vi "Check validate frequencies.vi"(8 "Check Delta Amplitude":bool[](array[boolean]), 9 "Check Amplitude":bool[](array[boolean]), 11 "Frequencies Array":dbl[](array[numeric])) -> (0 "variance":dbl format="%0.2f", 1 "Standard deviation %":dbl, 2 "standard deviation":dbl format="%0.2f", 3 "Mean frequency":dbl format="%0.2f")   [LabVIEW 2014]
uses:
  <vilib>/Analysis/NI_AALBase.lvlib
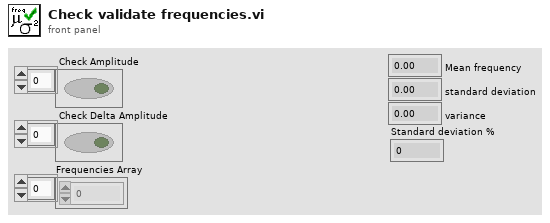
[diagram p1: front panel]
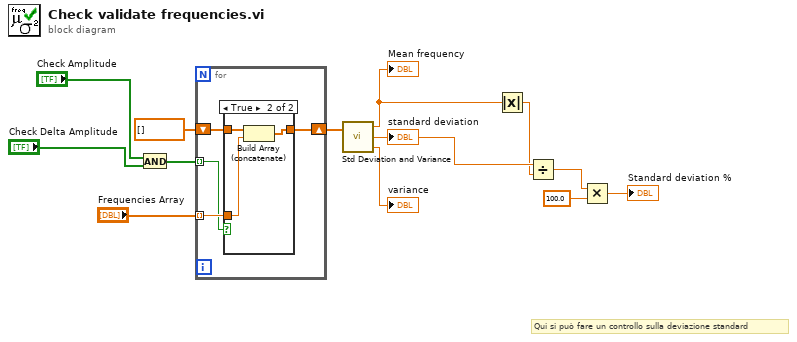
[diagram p0: block diagram]
diagram:
  # "Qui si può fare un controllo sulla deviazione standard"
  n1 = And(x="Check Amplitude", y="Check Delta Amplitude") -> (x .and. y?=w10:bool[])
  n2 = for {
    tunnel: "Frequencies Array" -> [w16] mode=indexing
    tunnel: w10 -> [w15] mode=indexing
    shift-right: [w14] -> w8
    shift-left: dbl[] [] ("Frequencies Array 2") -> [w17]
    n3 = case shown="True" w15 {
      tunnel: w17 -> [w18 w21]
      tunnel: w16 -> [_ w20]
      tunnel: [w18 w19] -> w14
      frame False {
      }
      frame True {
        n4 = Build Array (concatenate)(w21, w20) -> (w19:dbl[])
      }
    }
  }
  n5 = call <vilib>:"Std Deviation and Variance.vi"("X"=w8) -> ("mean"=w5:dbl, "standard deviation"=w6:dbl, "variance"=→"variance":dbl)  [unwired: 1 in]
  "Mean frequency" <- w5
  "standard deviation" <- w6
  n6 = Absolute Value(x=w5) -> (abs(x)=w4:dbl)
  n7 = Divide(x=w6, y=w4) -> (x/y=w3:dbl)
  n8 = Multiply(x=w3, y=100.0) -> (x*y=→"Standard deviation %":dbl)
